vi "Get status Response.vi"(8 "error in (no error)":errorcluster, 11 "Simulado in":refnum<class "Simulado.lvclass">) -> (0 "error out":errorcluster, 2 "Response":string, 3 "Simulado out":refnum<class "Simulado.lvclass">)   [LabVIEW 2020, in "Simulado.lvclass"]
uses:
  Simulado.lvclass
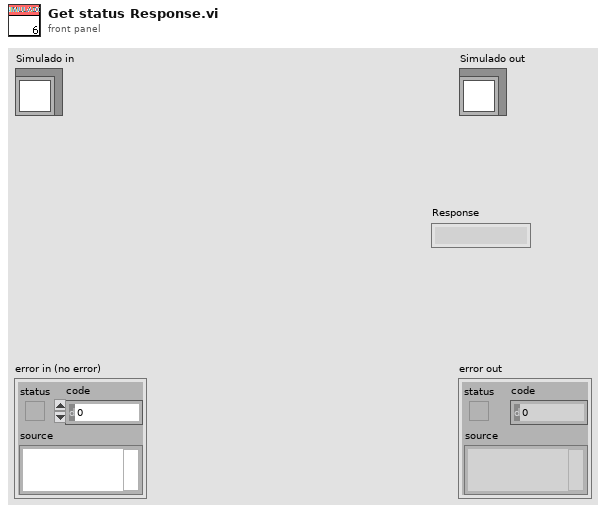
[diagram p1: front panel]
types:
  T1 = enum16{"reset parameters", "Get parameters", "Set parameter"}
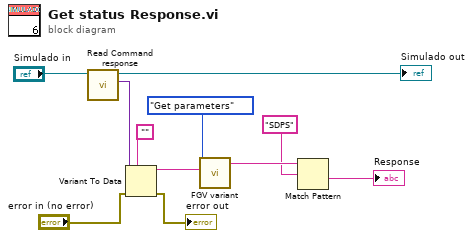
[diagram p0: block diagram]
diagram:
  n1 = call-dynamic "Read Command response.vi"("Simulado in"="Simulado in") -> ("Command response"=w9:variant, "Simulado out"=→"Simulado out":refnum<class "Simulado.lvclass">)  [unwired: 8 in, 1 out]
  n2 = Variant To Data(error in="error in (no error)", type="", Variant=w9) -> (data=w5:string, error out=→"error out":errorcluster)
  n3 = call "FGV variant.vi"("Command"=w5, "Functions"=T1."Get parameters") -> ("Response retrieved"=w2:string)  [unwired: 8 in, 1 out]
  n4 = Match Pattern(string=w2, regular expression="SDPS") -> (after substring=→"Response":string)  [unwired: 1 in, 3 out]
